vi "FGPA Sorting_PulseWidt.vi"() -> ()   [LabVIEW 2016]
uses:
  <vilib>/Analysis/baseanly.llb/Mean (DBL).vi
  <vilib>/FPGAPlugInAG/PCIe-7841R/niLvFpga_Open_PCIe-7841R.vi
  <vilib>/rvi/interface/common/dynamic/niFpgaDynamicAddResources.vi
  <vilib>/FPGAPlugInAG/Dynamic/niLvFpga_Reset_Dynamic.vi
  <vilib>/rvi/interface/common/niFpgaWaitOnOcc.vi
  <vilib>/Utility/error.llb/Error Cluster From Error Code.vi
  <vilib>/FPGAPlugInAG/Dynamic/niLvFpga_Run_Dynamic.vi
  <vilib>/rvi/Analysis/host/Private/Sample Rate To Loop Time (ticks).vi
  <vilib>/rvi/errors/niLvFpgaAdjustHostInterfaceError.vi
  <vilib>/FPGAPlugInAG/Dynamic/niLvFpga_Close_Dynamic.vi
  <vilib>/rvi/interface/nirviOpenFPGA/nirviOpenFPGA.xnode
  FPGA Bitfiles/FPGASortingWidth_FPGATarget_ReadAnalog3Pulse_hUFl5RTEBKk.lvbitx
  ReadAnalog3_PulseWidt.vi
  <vilib>/rvi/interface/nirviMethod/nirviMethod.xnode
  <vilib>/rvi/interface/nirviReadWriteControl/nirviReadWriteControl.xnode
  <vilib>/rvi/interface/nirviCloseFPGA/nirviCloseFPGA.xnode
  <vilib>/rvi/interface/Simulation/niFpgaSimulationCallBeginRW.vi
  <vilib>/rvi/Analysis/host/Public/NI_FpgaMspHost.lvlib
  <vilib>/rvi/errors/niLvFpgaMergeErrorWithErrorCode.vi
  <vilib>/Analysis/NI_AAL_SigProc.lvlib
  <vilib>/Analysis/NI_AALPro.lvlib
  <vilib>/Analysis/NI_AALBase.lvlib
  <vilib>/FPGAPlugInAG/Dynamic/niLvFpga_ConfigureFifo_Dynamic.vi
  <vilib>/FPGAPlugInAG/Dynamic/niLvFpga_ReadFifo_Dynamic.vi
  NiFpgaLv.dll
panel:
  in  "Boolean":bool
  out "Read Interval":i32
  out "XY Graph 2":cluster{u32[], "Array":dbl[]}(graph)
  in  "Noise Level":dbl=0.2
  out "Fraction Sorted":dbl
  out "Sorted Droplets":i16
  out "Total Droplets":i32
  out "Droplet Rate":dbl format="%0.2f"
  in  "PMT Voltage":dbl(slide) scale=0.0..1.25
  out "Filename Out":path
  in  "Save Histogram":bool caption="Enable"
  in  "Add":bool
  in  "Reset":bool
  out "Cumulative Histogram":T1(graph)
  out "Outside":cluster{"total":i32, "below":i32, "above":i32}
  in  "Bins":i32=1000
  in  "Min Signal":dbl=5.5 format="%0.2f"
  in  "Max Signal":dbl format="%0.2f"
  out "XY Graph":cluster{dbl[], "Amplitudes":dbl[]}[](graph)
  in  "Peak Width":i32=3 min=3
  in  "Peak Minimum":dbl=5.0 format="%0.2f"
  in  "Sorting Threshold":dbl=10.0
  out "Event":bool
  out "Sample Rate":dbl format="%#_6p"
  in  "FPGA Loop Rate (Hz)":dbl=50000.0 format="%#_6p"
  in  "stop":bool
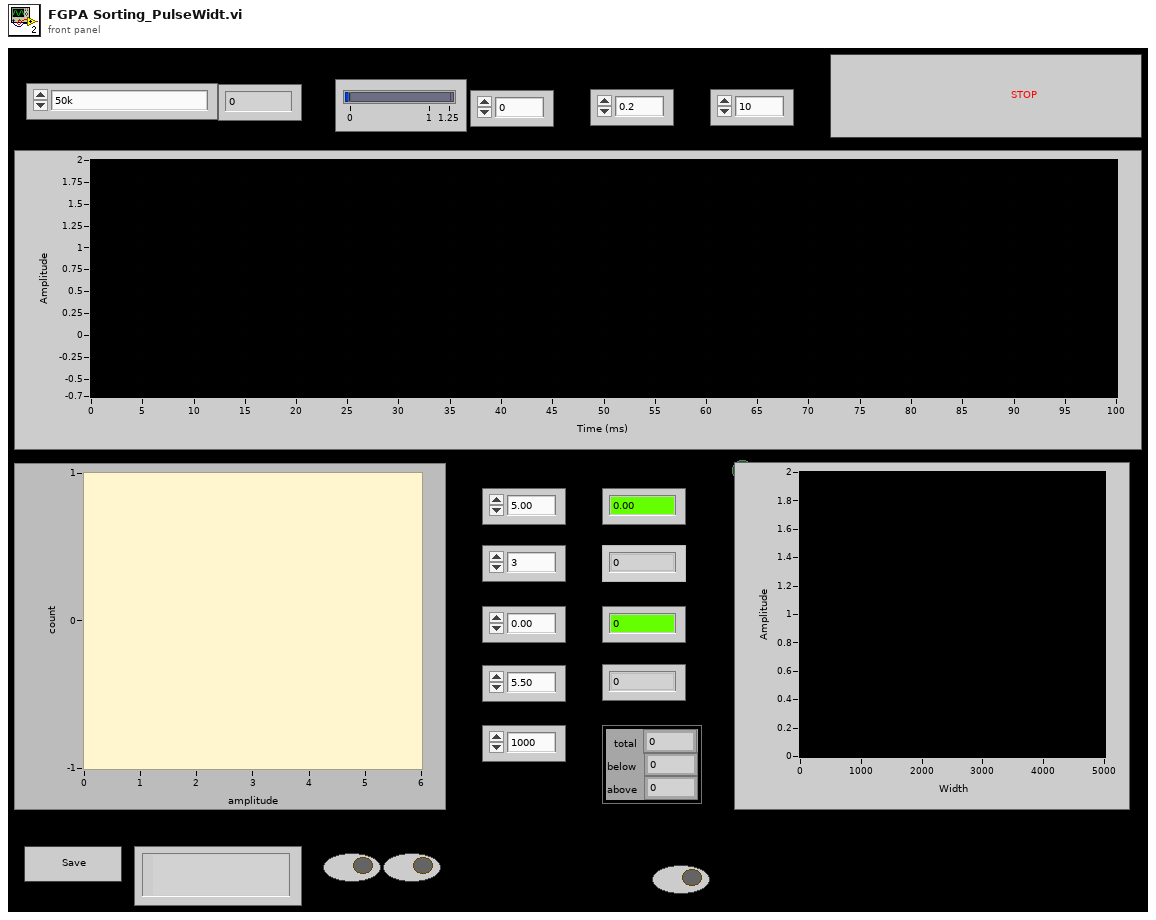
[diagram p1: front panel]
types:
  T1 = cluster{"X Values":dbl[], "Histogram: h(x)":i32[]}
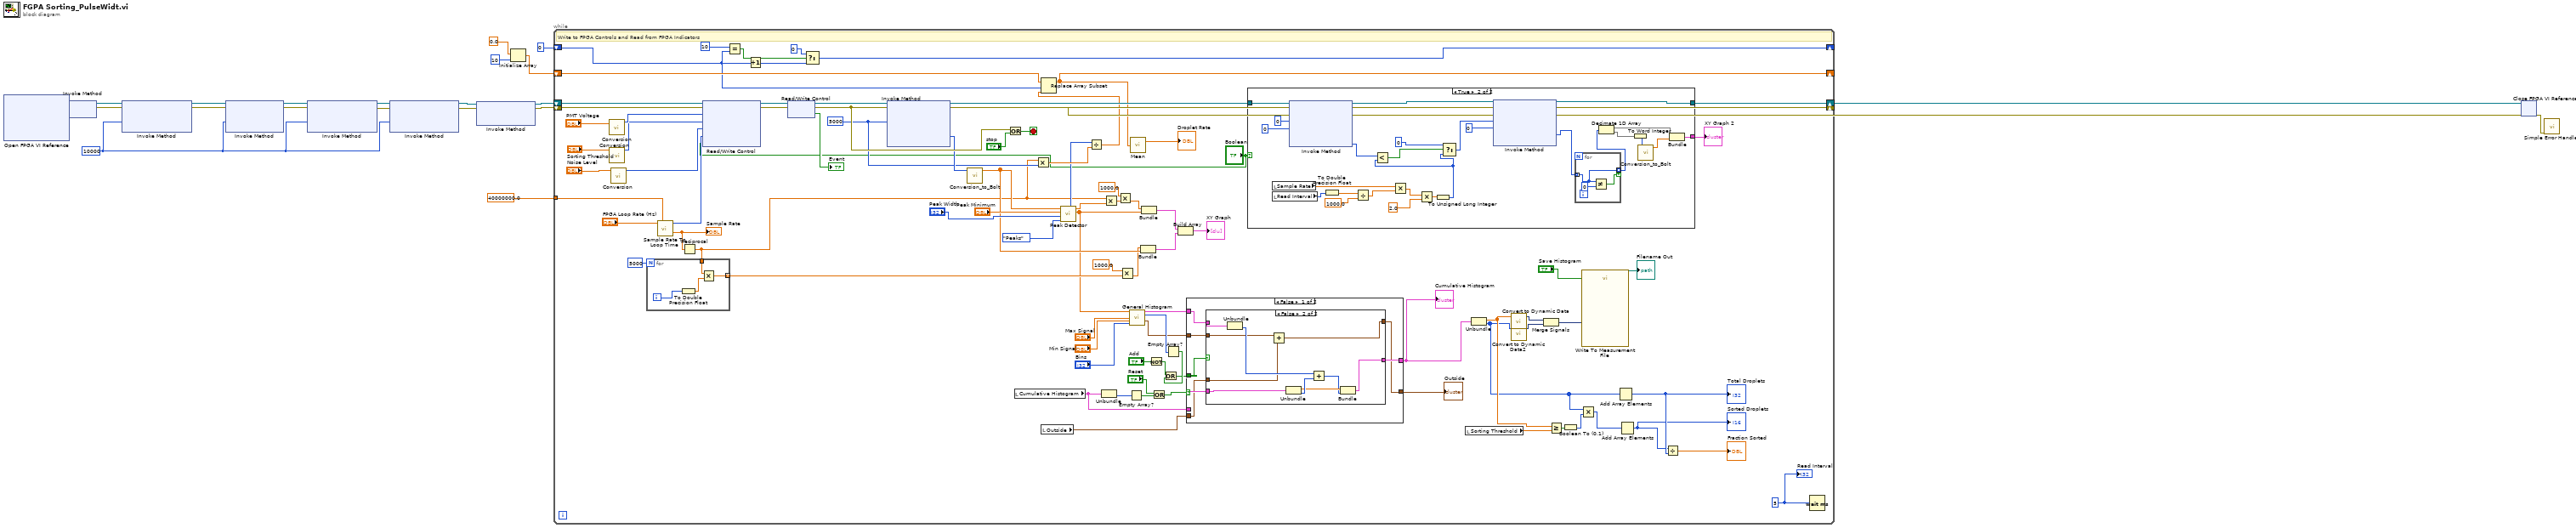
[diagram p0: block diagram]
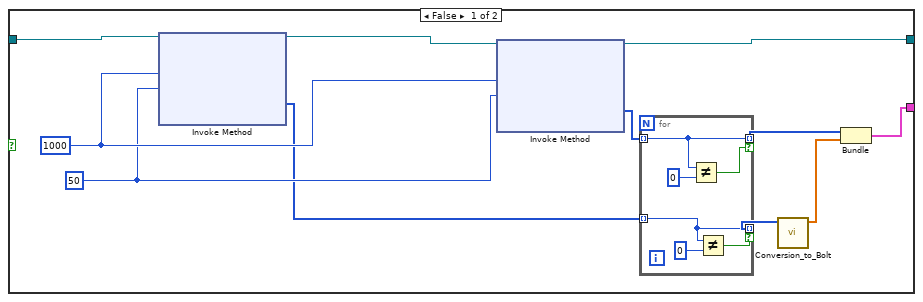
[diagram p2: hidden frame]
diagram:
  w1 = u32 10000 ("Requested Depth")
  n1 = xnode "Open FPGA VI Reference"() -> ("FPGA VI Reference Out"=w20:refnum<k20>, "error out"=w10:errorcluster)  [unwired: 2 in]
  n2 = xnode "Invoke Method"("FPGA VI Reference In"=w20, "error in"=w10) -> ("FPGA VI Reference Out"=w11:refnum<k20>, "error out"=w9:errorcluster)
  n3 = xnode "Invoke Method"("FPGA VI Reference In"=w11, "error in"=w9, "Requested Depth"=w1) -> ("FPGA VI Reference Out"=w15:refnum<k20>, "error out"=w13:errorcluster)  [unwired: 1 out]
  n4 = xnode "Invoke Method"("FPGA VI Reference In"=w15, "Requested Depth"=w1) -> ("FPGA VI Reference Out"=w4:refnum<k20>)  [unwired: 1 in, 2 out]
  n5 = xnode "Invoke Method"("FPGA VI Reference In"=w4, "Requested Depth"=w1) -> ("FPGA VI Reference Out"=w3:refnum<k20>)  [unwired: 1 in, 2 out]
  n6 = xnode "Invoke Method"("FPGA VI Reference In"=w3, "Requested Depth"=w1) -> ("FPGA VI Reference Out"=w2:refnum<k20>)  [unwired: 1 in, 2 out]
  n7 = xnode "Invoke Method"("FPGA VI Reference In"=w2, "error in"=w13) -> ("FPGA VI Reference Out"=w14:refnum<k20>, "error out"=w12:errorcluster)  [unwired: 1 in]
  n8 = Initialize Array(0.0 ("element"), 10 ("dimension size")) -> (w7:dbl[])
  n9 = while {
    shift-right: [w29] -> w18
    shift-left: w12 -> [w105]
    shift-right: [w24] -> w19
    shift-left: w14 -> [w108]
    tunnel: 40000000.0 ("FPGA clock rate (Hz)") -> [w103]
    shift-right: [w51] -> _
    shift-left: w7 -> [w52]
    shift-right: [w39] -> _
    shift-left: 0 ("dimension size") -> [w40]
    stop <- w104 stop-if-true
    w23 = 5
    w74 = u32 5000 ("Number of Elements")
    # "Write to FPGA Controls and Read from FPGA Indicators"
    n10 = call "Conversion.vi"("Sorting Threshold"="PMT Voltage") -> ("Numeric 2"=w33:i16)  [unwired: 10 in]
    n11 = call "Conversion.vi"("Sorting Threshold"="Sorting Threshold") -> ("Numeric 2"=w32:i16)  [unwired: 10 in]
    n12 = call "Conversion.vi"("Sorting Threshold"="Noise Level") -> ("Numeric 2"=w30:i16)  [unwired: 10 in]
    n13 = call-poly <vilib>:"Sample Rate To Loop Time.vi"("sample rate (S/s)"="FPGA Loop Rate (Hz)", "FPGA clock rate (Hz)"=w103) -> ("count (ticks/S)"=w55:u32, "actual sample rate (S/s)"=w90:dbl)  [unwired: 11 in, 1 out]
    "Sample Rate" <- w90
    n14 = Reciprocal(x=w90) -> (1/x=w71:dbl)
    n15 = for {
      N: 5000 -> [_]
      tunnel: w71 -> [w178]
      tunnel: [w176] -> w89 mode=indexing
      i -> [w179]
      n16 = To Double Precision Float(number=w179) -> (double precision float=w177:dbl)
      n17 = Multiply(x=w178, y=w177) -> (x*y=w176:dbl)
    }
    n18 = xnode "Read/Write Control"("FPGA VI Reference In"=w108, "error in"=w105, "PMT Voltage"=w33, "Sorting Threshold"=w32, "Noise Level"=w30, "Loop Period (ticks)"=w55, "Array"="Boolean") -> ("FPGA VI Reference Out"=w107:refnum<k20>, "error out"=w106:errorcluster)
    n19 = Equal?(x=10, y=w40) -> (x = y?=w42:bool)
    n20 = Increment(x=w40) -> (x+1=w41:i32)
    n21 = xnode "Read/Write Control"("FPGA VI Reference In"=w107, "error in"=w106) -> ("FPGA VI Reference Out"=w102:refnum<k20>, "error out"=w99:errorcluster, "Event"=→"Event":bool)
    n22 = Select(t=0, s=w42, f=w41) -> (s? t:f=w39:i32)
    n23 = xnode "Invoke Method"("FPGA VI Reference In"=w102, "error in"=w99, "Number of Elements"=w74) -> ("FPGA VI Reference Out"=w56:refnum<k20>, "error out"=w29:errorcluster, "Data"=w84:i16[])  [unwired: 1 in, 1 out]
    n24 = call "Conversion_to_Bolt.vi"("Data"=w84) -> ("Array"=w94:dbl[])  [unwired: 10 in]
    n25 = Or(x=w99, y="stop") -> (x .or. y?=w104:bool)
    n26 = local read "Cumulative Histogram"() -> (w58:T1)
    n27 = Multiply(x=w71, y=w74) -> (x*y=w73:dbl)
    n28 = local read "Outside"() -> (w57:cluster{"total":i32, "below":i32, "above":i32})
    n29 = call <vilib>:"Peak Detector.vi"("peaks/valleys"=enum32{"Peaks", "Valleys"}."Peaks", "width"="Peak Width", "threshold"="Peak Minimum", "X"=w94) -> ("Amplitudes"=w81:dbl[], "Locations"=w83:dbl[], "# found"=w72:i32)  [unwired: 3 in, 2 out]
    n30 = Divide(x=w72, y=w73) -> (x/y=w53:dbl)
    n31 = Replace Array Subset(array=w52, new element=w53, index=w40) -> (w51:dbl[])
    n32 = Unbundle(w58) -> ("Histogram: h(x)"=w65:i32[])  [unwired: 1 out]
    n33 = Multiply(x=w71, y=w83) -> (x*y=w80:dbl[])
    n34 = Multiply(x=1000.0, y=w80) -> (x*y=w28:dbl[])
    n35 = Multiply(x=1000.0, y=w89) -> (x*y=w25:dbl[])
    n36 = Empty Array?(array=w65) -> (empty?=w66:bool)
    n37 = call <vilib>:"General Histogram.vi"("X"=w81, "max"="Max Signal", "min"="Min Signal", "# bins"="Bins") -> ("Histogram Graph"=w61:T1, "Histogram"=w62:i32[], "# outside"=w60:cluster{"total":i32, "below":i32, "above":i32})  [unwired: 7 in, 2 out]
    n38 = call-poly <vilib>:"Mean.vi"("X"=w51) -> ("mean"=→"Droplet Rate":dbl)  [unwired: 1 out]
    n39 = Bundle(w25, "Array"=w94) -> (w88:cluster{dbl[], "Array":dbl[]})  [unwired: 1 in]
    n40 = Bundle(w28, "Amplitudes"=w81) -> (w82:cluster{dbl[], "Amplitudes":dbl[]})  [unwired: 1 in]
    n41 = Not(x="Add") -> (.not. x?=w70:bool)
    n42 = Or(x="Reset", y=w66) -> (x .or. y?=w67:bool)
    n43 = Empty Array?(array=w62) -> (empty?=w69:bool)
    n44 = Or(x=w70, y=w69) -> (x .or. y?=w68:bool)
    n45 = Build Array(w82, w88) -> (→"XY Graph":cluster{dbl[], "Array":dbl[]}[])
    n46 = case shown="False" w67 {
      tunnel: [w161 w175] -> w59
      tunnel: w68 -> [w160 _]
      tunnel: [w159 w174] -> w48
      tunnel: w61 -> [w158 w175]
      tunnel: w60 -> [w157 w174]
      tunnel: w58 -> [w156 _]
      tunnel: w57 -> [w155 _]
      frame False {
        n47 = case shown="False" w160 {
          tunnel: [w163 w170] -> w161
          tunnel: [w162 w169] -> w159
          tunnel: w158 -> [_ w168]
          tunnel: w157 -> [_ w166]
          tunnel: w156 -> [w163 w165]
          tunnel: w155 -> [w162 w164]
          frame True {
          }
          frame False {
            n48 = Unbundle(w168) -> ("Histogram: h(x)"=w167:i32[])  [unwired: 1 out]
            n49 = Add(x=w166, y=w164) -> (x+y=w169:cluster{"total":i32, "below":i32, "above":i32})
            n50 = Unbundle(w165) -> ("X Values"=w172:dbl[], "Histogram: h(x)"=w173:i32[])
            n51 = Add(x=w167, y=w173) -> (x+y=w171:i32[])
            n52 = Bundle("X Values"=w172, w171) -> (w170:cluster{"X Values":dbl[], i32[]})  [unwired: 1 in]
          }
        }
      }
      frame True {
      }
    }
    "Outside" <- w48
    "Cumulative Histogram" <- w59
    n53 = case shown="True" "Boolean" {
      tunnel: w56 -> [w119 w151]
      tunnel: [w117 w149] -> w24
      tunnel: [w113 w133] -> w22
      frame False {
        w115 = 50
        w116 = u32 1000 ("Number of Elements")
        n54 = xnode "Invoke Method"("FPGA VI Reference In"=w119, "Number of Elements"=w116, "Timeout (ms)"=w115) -> ("FPGA VI Reference Out"=w118:refnum<k20>, "Data"=w111:i16[])  [unwired: 1 in, 2 out]
        n55 = xnode "Invoke Method"("FPGA VI Reference In"=w118, "Number of Elements"=w116, "Timeout (ms)"=w115) -> ("FPGA VI Reference Out"=w117:refnum<k20>, "Data"=w110:u32[])  [unwired: 1 in, 2 out]
        n56 = for {
          tunnel: [w124] -> w112 mode=indexing if=w125
          tunnel: w111 -> [w124] mode=indexing
          tunnel: w110 -> [w121] mode=indexing
          tunnel: [w121] -> w109 mode=indexing if=w120
          n57 = Not Equal?(x=w121, y=u32 0) -> (x != y?=w120:bool)
          n58 = Not Equal?(x=w124, y=i16 0) -> (x != y?=w125:bool)
        }
        n59 = call "Conversion_to_Bolt.vi"("Data"=w112) -> ("Array"=w114:dbl[])  [unwired: 10 in]
        n60 = Bundle(w109, "Array"=w114) -> (w113:cluster{u32[], "Array":dbl[]})  [unwired: 1 in]
      }
      frame True {
        n61 = local read "Sample Rate"() -> (w144:dbl)
        n62 = local read "Read Interval"() -> (w147:i32)
        n63 = xnode "Invoke Method"("FPGA VI Reference In"=w151, "Number of Elements"=u32 0, "Timeout (ms)"=0) -> ("FPGA VI Reference Out"=w150:refnum<k20>, "Elements Remaining"=w137:u32)  [unwired: 1 in, 2 out]
        n64 = To Double Precision Float(number=w147) -> (double precision float=w146:dbl)
        n65 = Divide(x=w146, y=1000.0) -> (x/y=w143:dbl)
        n66 = Multiply(x=w144, y=w143) -> (x*y=w142:dbl)
        n67 = Multiply(x=w142, y=2.0) -> (x*y=w140:dbl)
        n68 = To Unsigned Long Integer(number=w140) -> (unsigned 32bit integer=w135:u32)
        n69 = Less?(x=w137, y=w135) -> (x < y?=w136:bool)
        n70 = Select(t=u32 0, s=w136, f=w135) -> (s? t:f=w128:u32)
        n71 = xnode "Invoke Method"("FPGA VI Reference In"=w150, "Number of Elements"=w128, "Timeout (ms)"=0) -> ("FPGA VI Reference Out"=w149:refnum<k20>, "Data"=w127:i32[])  [unwired: 1 in, 2 out]
        n72 = for {
          tunnel: w127 -> [w154] mode=indexing
          tunnel: [w154] -> w126 mode=indexing if=w152
          n73 = Not Equal?(x=w154, y=0) -> (x != y?=w152:bool)
        }
        n74 = Decimate 1D Array(w126) -> (w130:i32[], w131:i32[])
        n75 = To Word Integer(number=w131) -> (16bit integer=w132:i16[])
        n76 = call "Conversion_to_Bolt.vi"("Data"=w132) -> ("Array"=w129:dbl[])  [unwired: 10 in]
        n77 = Bundle(w130, "Array"=w129) -> (w133:cluster{i32[], "Array":dbl[]})  [unwired: 1 in]
      }
    }
    "XY Graph 2" <- w22
    n78 = local read "Sorting Threshold"() -> (w49:dbl)
    n79 = Unbundle(w59) -> ("X Values"=w38:dbl[], "Histogram: h(x)"=w37:i32[])
    n80 = call "Convert to Dynamic Data2"("Array"=w37) -> ("Dynamic Data Type"=w77:dynamicdata)  [unwired: 3 in]
    n81 = call "Convert to Dynamic Data"("Array"=w38) -> ("Dynamic Data Type"=w79:dynamicdata)  [unwired: 3 in]
    n82 = Merge Signals(w79, w77) -> (w78:dynamicdata)
    n83 = Greater Or Equal?(x=w38, y=w49) -> (x >= y?=w35:bool[])
    n84 = Boolean To (0,1)(Boolean=w35) -> (0, 1=w34:i16[])
    n85 = Multiply(x=w37, y=w34) -> (x*y=w36:i32[])
    n86 = call "Write To Measurement File"("Signals"=w78, "Enable"="Save Histogram") -> ("Filename Out"=→"Filename Out":path)  [unwired: 15 in, 2 out]
    n87 = Add Array Elements(numeric array=w37) -> (sum=w47:i32)
    "Total Droplets" <- w47
    n88 = Add Array Elements(numeric array=w36) -> (sum=w46:i32)
    "Sorted Droplets" <- w46
    n89 = Divide(x=w46, y=w47) -> (x/y=→"Fraction Sorted":dbl)
    n90 = Wait (ms)(milliseconds to wait=w23) -> ()  [unwired: 1 out]
    "Read Interval" <- w23
  }
  n91 = xnode "Close FPGA VI Reference"("FPGA VI Reference In"=w19, "error in"=w18) -> ("error out"=w17:errorcluster)
  n92 = call <vilib>:"Simple Error Handler.vi"("error in (no error)"=w17) -> ()  [unwired: 4 in, 5 out]
